vi "Init Serial (Direct).vi"(7 "Error Checking (Full)":T2=enum."Full", 8 "error in (no error)":errorcluster, 10 "Baud (115200)":u32=115200, 11 "VISA resource name in":refnum<visa-resource-name>) -> (0 "error out":errorcluster, 3 "VisaComms out":refnum<class "VisaComms.lvclass">, 5 "Identity":T1)   [LabVIEW 2024, in "CTI.lvlib" / "VisaComms.lvclass"]
doc: "Creates a Visa Communications instance for interacting with CTI firmware with SCPI based communications.\n\nUsing this (Direct) version of VisaComms avoids the extra layers of code that exist in the (Session) version so that it can be quicker and easier to see and debug the lower level communications with the device at the expense of the additional functionality provided by sessions.\n\nThe (Session) version of the Init VI should be used if any of the following functionality is desired:\n- Checks for valid pin mappings\n- Checks for conflicting pin usage\n- Built-in support for usage in parallel code\n- Usage of peripheral libraries that rely on Sessions"
uses:
  VisaComms.lvclass
  Error Reporting.ctl
  Identity.ctl
  <vilib>/Instr/_visa.llb/VISA Open Access Mode.ctl
  VisaComms.lvclass/VisaComms.ctl
  <vilib>/Instr/_visa.llb/VISA Configure Serial Port (Instr).vi
  CTI.lvlib
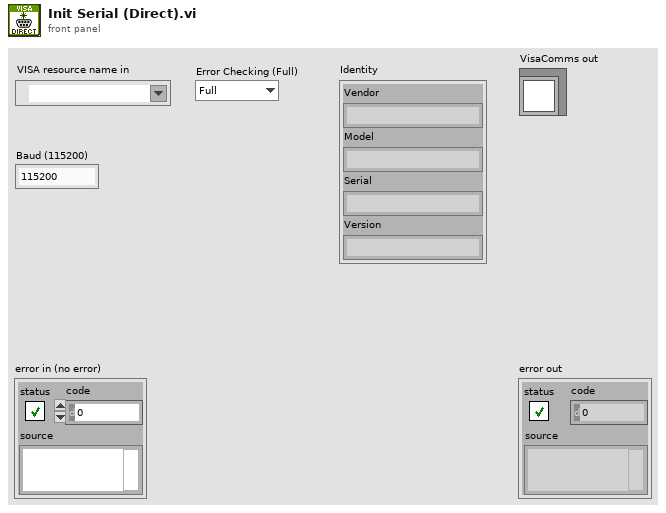
[diagram p1: front panel]
types:
  T1 = typedef "CTI.lvlib/Identity.ctl" = cluster{"Vendor":string, "Model":string, "Serial":string, "Version":string}
  T2 = typedef "CTI.lvlib/Error Reporting.ctl" = enum16{"Minimal", "Moderate", "Full"}
  T3 = typedef "VISA Open Access Mode.ctl" = u32
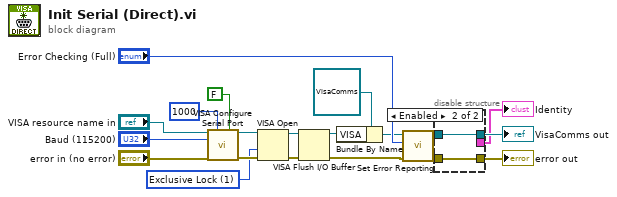
[diagram p0: block diagram]
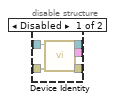
[diagram p2: hidden frame]
diagram:
  w14 = T3 1 items=["VISA Defaults"=0, "Exclusive Lock"=1, "Load Configured Settings"=4] ("Access Mode")
  n1 = call-poly "VISA Configure Serial Port"("VISA resource name"="VISA resource name in", "timeout (10sec)"=u32 1000, "Enable Termination\nChar (T)"=FALSE ("Enable Termination\nChar (T)"), "baud rate (9600)"="Baud (115200)", "error in (no error)"="error in (no error)") -> ("VISA resource name out"=w15:refnum<visa-resource-name>, "error out"=w16:errorcluster)  [unwired: 9 in]
  n2 = VISA Open(access mode=w14, error in (no error)=w16, VISA resource name=w15) -> (VISA resource name=w12:refnum<visa-resource-name>, error out=w2:errorcluster)  [unwired: 2 in]
  n3 = VISA Flush I/O Buffer(VISA resource name=w12, error in (no error)=w2) -> (VISA resource name out=w3:refnum<visa-resource-name>, error out=w1:errorcluster)  [unwired: 1 in]
  n4 = Bundle By Name(cluster=refnum<class "VisaComms.lvclass"> refnum ("VisaComms in"), "VISA"=w3) -> (w13:refnum<class "VisaComms.lvclass">)
  n5 = call-dynamic "Set Error Reporting.vi"("error in (no error)"=w1, "Error Reporting"="Error Checking (Full)", "VisaComms in"=w13) -> ("error out"=w9:errorcluster, "VisaComms out"=w7:refnum<class "VisaComms.lvclass">)  [unwired: 7 in]
  n6 = disable-structure shown="Enabled" {
    disable-tunnel: w9 -> [w25 w26]
    disable-tunnel: [w24 w26] -> w8
    disable-tunnel: w7 -> [w23 w27]
    disable-tunnel: [w22 w27] -> w6
    disable-tunnel: [w21 _] -> w5
    frame Disabled {
      n7 = call-dynamic "Device Identity.vi"("error in (no error)"=w25, "VisaComms in"=w23) -> ("error out"=w24:errorcluster, "Identity"=w21:T1, "VisaComms out"=w22:refnum<class "VisaComms.lvclass">)  [unwired: 7 in]
    }
    frame Enabled {
    }
  }
  "error out" <- w8
  "VisaComms out" <- w6
  "Identity" <- w5
